vi "MGI Interpolate 1D Array Extended.vi"(2 "Fractional X":dbl, 3 "Y Value[]":dbl[](array[numeric])) -> (0 "ExtendedY":dbl)   [LabVIEW 2019]
doc: "Extended version of Interpolate 1D Array which can extrapolate outside of the array bounds. Linear extension based on the first or last two array elements is used for out of range values.\n\nAuthored by David A. Moore\nsupport@mooregoodideas.com\nwww.mooregoodideas.com\n\nCopyright (c) 2010, Moore Good Ideas, Inc.\n\nAll rights reserved.\n\nRedistribution and use in source and binary forms, with or without modification, are permitted provided that the following conditions are met:\n\n * Redistributions of source code must retain the above copyright notice, this list of conditions and the following disclaimer.\n * Redistributions in binary form must reproduce the above copyright notice, this list of conditions and the following disclaimer in the documentation and/or other materials provided with the distribution.\n * Neither the name of Moore Good Ideas, Inc. nor the names of its contributors may be used to endorse or promote products derived from this software without specific prior written permission.\n\nTHIS SOFTWARE IS PROVIDED BY THE COPYRIGHT HOLDERS AND CONTRIBUTORS \"AS IS\" AND ANY EXPRESS OR IMPLIED WARRANTIES, INCLUDING, BUT NOT LIMITED TO, THE IMPLIED WARRANTIES OF MERCHANTABILITY AND FITNESS FOR A PARTICULAR PURPOSE ARE DISCLAIMED. IN NO EVENT SHALL THE COPYRIGHT OWNER OR CONTRIBUTORS BE LIABLE FOR ANY DIRECT, INDIRECT, INCIDENTAL, SPECIAL, EXEMPLARY, OR CONSEQUENTIAL DAMAGES (INCLUDING, BUT NOT LIMITED TO, PROCUREMENT OF SUBSTITUTE GOODS OR SERVICES; LOSS OF USE, DATA, OR PROFITS; OR BUSINESS INTERRUPTION) HOWEVER CAUSED AND ON ANY THEORY OF LIABILITY, WHETHER IN CONTRACT, STRICT LIABILITY, OR TORT (INCLUDING NEGLIGENCE OR OTHERWISE) ARISING IN ANY WAY OUT OF THE USE OF THIS SOFTWARE, EVEN IF ADVISED OF THE POSSIBILITY OF SUCH DAMAGE."
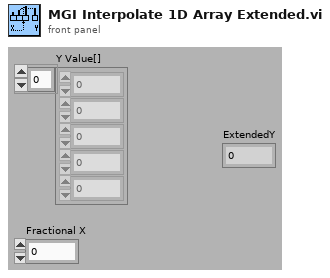
[diagram p1: front panel]
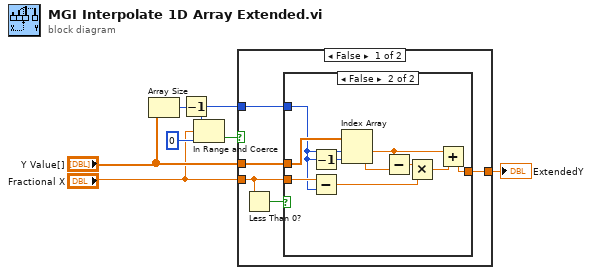
[diagram p0: block diagram]
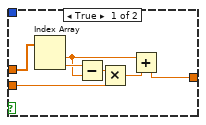
[diagram p2: hidden frame]
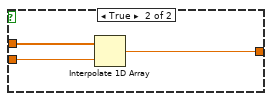
[diagram p3: hidden frame]
diagram:
  n1 = Array Size(array="Y Value[]") -> (size(s)=w4:i32)
  n2 = Decrement(x=w4) -> (x-1=w6:i32)
  n3 = In Range and Coerce(upper limit=w6, x="Fractional X", lower limit=0) -> (In Range?=w7:bool)  [unwired: 1 out]
  n4 = case shown="False" w7 {
    tunnel: [w8 w32] -> w3
    tunnel: "Y Value[]" -> [w10 w31]
    tunnel: "Fractional X" -> [w11 w30]
    tunnel: w6 -> [w9 _]
    frame False {
      n5 = Less Than 0?(x=w11) -> (x < 0?=w12:bool)
      n6 = case shown="False" w12 {
        tunnel: w11 -> [w16 w22]
        tunnel: w10 -> [w19 w29]
        tunnel: w9 -> [_ w21]
        tunnel: [w13 w24] -> w8
        frame True {
          n7 = Index Array(array=w19) -> (element #1=w14:dbl, element #2=w18:dbl)  [unwired: 2 in]
          n8 = Subtract(x=w18, y=w14) -> (x-y=w17:dbl)
          n9 = Multiply(x=w17, y=w16) -> (x*y=w15:dbl)
          n10 = Add(x=w14, y=w15) -> (x+y=w13:dbl)
        }
        frame False {
          n11 = Decrement(x=w21) -> (x-1=w23:i32)
          n12 = Subtract(x=w22, y=w21) -> (x-y=w20:dbl)
          n13 = Index Array(array=w29, index #1=w21, index #2=w23) -> (element #1=w25:dbl, element #2=w28:dbl)
          n14 = Subtract(x=w25, y=w28) -> (x-y=w27:dbl)
          n15 = Multiply(x=w27, y=w20) -> (x*y=w26:dbl)
          n16 = Add(x=w25, y=w26) -> (x+y=w24:dbl)
        }
      }
    }
    frame True {
      n17 = Interpolate 1D Array(1:w30, 2:w31) -> (0:w32:dbl)
    }
  }
  "ExtendedY" <- w3
